vi "StageLinear.vi"(0 "Axis":T1={"Serial port handle"="", "Axis"="", "Controller #"=0, "Min position"=0.0, "Max position"=0.0, "Min velocity"=0.0, "Max velocity"=0.0, "Firmware"="", "Device ID"=0, "Variable event"=refnum, "Variable ref"=refnum, "Resolution, usteps/step"=0, "Serial port semaphore"=refnum, "Joystick buttons"={"MinDir"=1, "MaxDir"=2, "MedSpeed"=5, "HighSpeed"=6}} {"Joystick buttons"."HighSpeed" min=1 max=25 step=1; "Joystick buttons"."MedSpeed" min=1 max=25 step=1; "Joystick buttons"."MaxDir" min=1 max=25 step=1; "Joystick buttons"."MinDir" min=1 max=25 step=1}, 2 "Joystick event":T4, 3 "Stop event":refnum<user-event>, 5 "error in":errorcluster={"status"=FALSE, "code"=1073676294, "source"="VISA Read in Zaber TLCM.lvclass:Command.vi:1820008->Zaber TLCM.lvclass:Get home position.vi->Zaber TLCM.lvclass:Get limits.vi->Zaber TLCM.lvclass:Join.vi->Swan probe.vi"}) -> (14 "Axis out":T1={"Serial port handle"="", "Axis"="", "Controller #"=0, "Min position"=0.0, "Max position"=0.0, "Min velocity"=0.0, "Max velocity"=0.0, "Firmware"="", "Device ID"=0, "Variable event"=refnum, "Variable ref"=refnum, "Resolution, usteps/step"=0, "Serial port semaphore"=refnum, "Joystick buttons"={"MinDir"=1, "MaxDir"=2, "MedSpeed"=5, "HighSpeed"=6}} {"Joystick buttons"."HighSpeed" min=1 max=25 step=1; "Joystick buttons"."MedSpeed" min=1 max=25 step=1; "Joystick buttons"."MaxDir" min=1 max=25 step=1; "Joystick buttons"."MinDir" min=1 max=25 step=1}, 19 "error out":errorcluster)   [LabVIEW 2017]
uses:
  Joystick events/Joystick event.ctl
  GenericDataEvent/GenericEvent.ctl
  Zaber.ctl
  ZaberVariables.ctl
panel:
  in  "Tab Control":enum32{"Joystick", "Keyboard"}(tab)
  in  "JoyLowVel":dbl=0.02 caption="Low velocity, mm/s" min=1e-07 max=25.0 step=0.01 format="%#.4f"
  in  "JoyMediumVel":dbl=1.0 caption="Medium velocity, mm/s" min=1e-07 max=25.0 step=0.01 format="%#.4f"
  in  "JoyHighVel":dbl=5.0 caption="High velocity, mm/s" min=1e-07 max=25.0 step=0.01 format="%#.4f"
  out "JoyMinDirection":i32=1 caption="Min direction" min=1 max=25 step=1
  out "JoyMaxDirection":i32=2 caption="Max direction" min=1 max=25 step=1
  out "JoyMediumVelocity":i32=5 caption="Max direction" min=1 max=25 step=1
  out "JoyHighVelocity":i32=6 caption="Max direction" min=1 max=25 step=1
  in  "BtnJogNegative":bool
  in  "BtnJogPositive":bool
  in  "JogStep":dbl=0.02 caption="Jog step, mm" min=1e-07 max=25.0 step=0.01 format="%#.4f"
  out "JoystickValue":i16
  in  "Readback loop":bool=TRUE
  out "Name":string
  in  "VelocitySp":dbl=0.19998779296875002 caption="Velocity, mm/s" min=0.0 max=25.40003175 format="%#.6f"
  out "VelocityRb":dbl=0.19998779296875002 caption="X position" min=0.0 max=25.0 format="%#.6f"
  in  "PositionSp":dbl caption="Position, mm" min=0.0 max=25.40003175 format="%#.6f"
  out "PositionRb":dbl=0.8111490000000001 caption="X position" min=0.0 max=25.0 format="%#.6f"
  out "MaxVelocity":dbl=26.0 caption="Max velocity, mm/s" format="%#.4f"
  out "MaxPositionRb":dbl=101.60003175000001 caption="Max position, mm" format="%#.4f"
  out "MinPositionRb":dbl caption="Min position, mm" format="%#.4f"
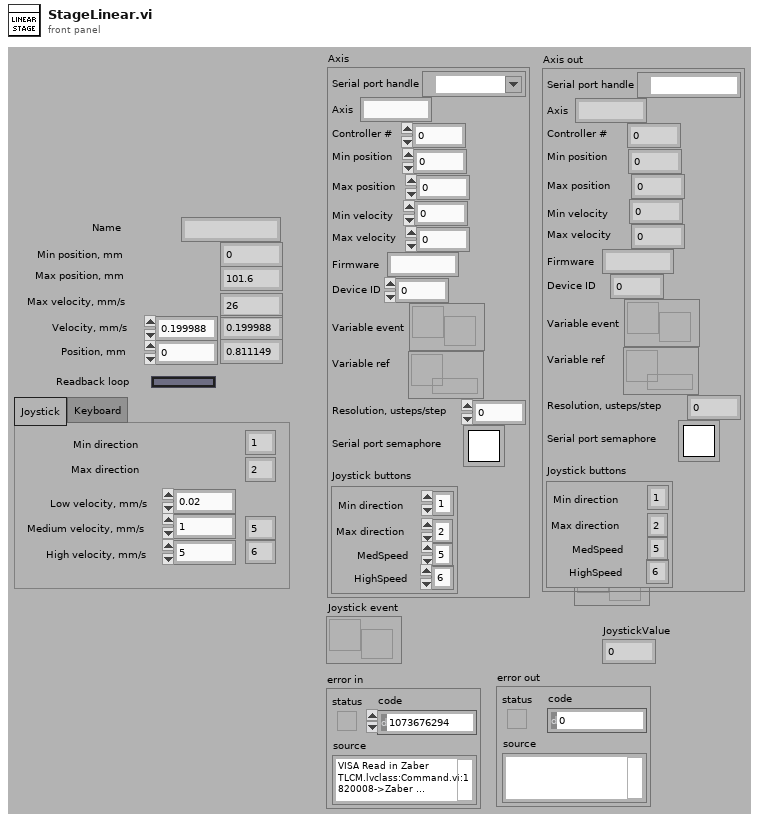
[diagram p1: front panel]
types:
  T1 = typedef "Zaber.ctl" = cluster{"Serial port handle":refnum<visa-resource-name>, "Axis":string, "Controller #":u8, "Min position":dbl, "Max position":dbl, "Min velocity":dbl, "Max velocity":dbl, "Firmware":string, "Device ID":i32, "Variable event":T2, "Variable ref":refnum<data-value>, "Resolution, usteps/step":i32, "Serial port semaphore":T3, "Joystick buttons":cluster{"MinDir":i32, "MaxDir":i32, "MedSpeed":i32, "HighSpeed":i32}}
  T2 = typedef "GenericEvent.ctl" = refnum<user-event>
  T3 = typedef "Semaphore RefNum" = refnum<k1>
  T4 = typedef "Joystick event.ctl" = refnum<user-event>
  T5 = cluster{"MinDir":i32, "MaxDir":i32, "MedSpeed":i32, "HighSpeed":i32}
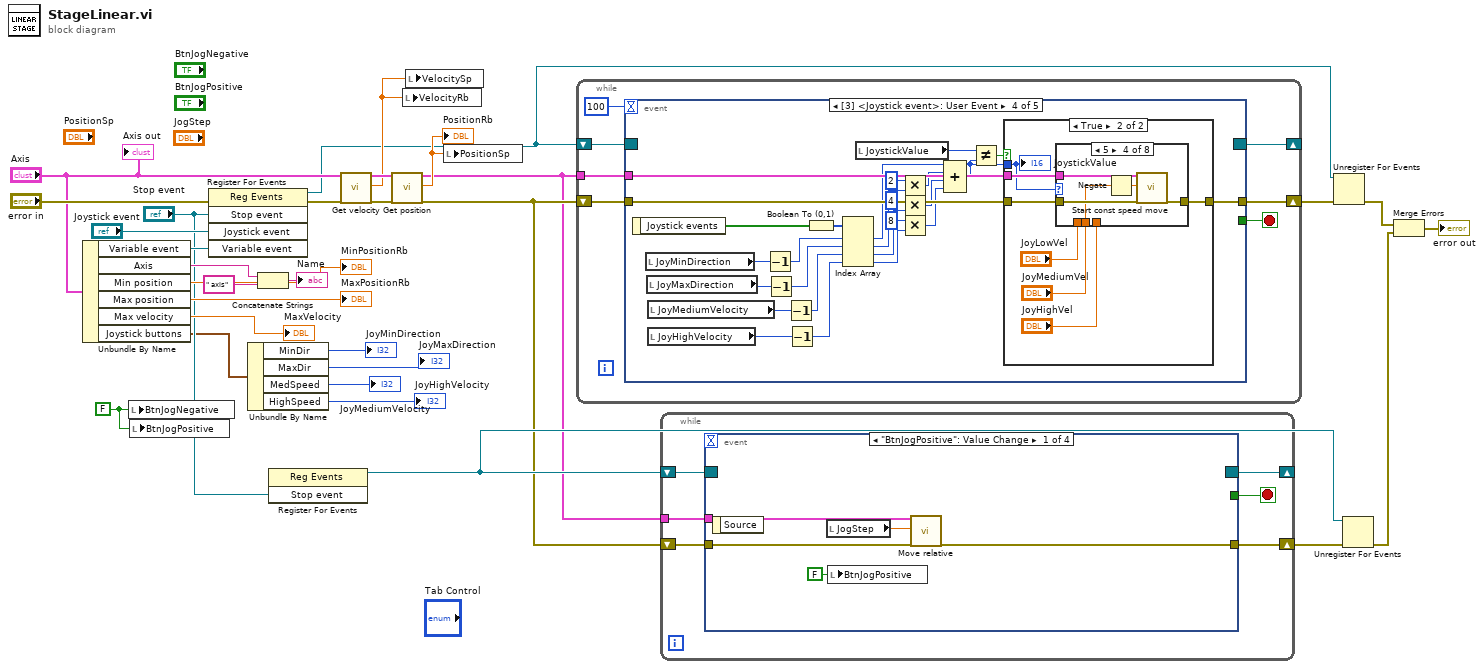
[diagram p0: block diagram]
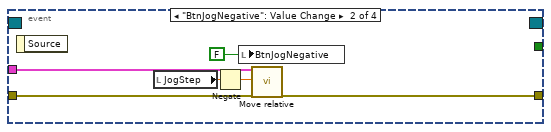
[diagram p2: hidden frame]
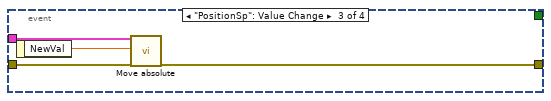
[diagram p3: hidden frame]
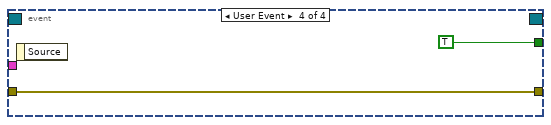
[diagram p4: hidden frame]
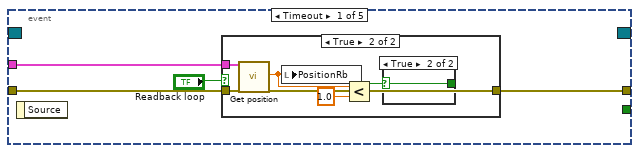
[diagram p5: hidden frame]
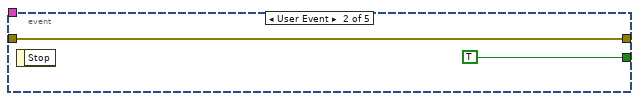
[diagram p8: hidden frame]
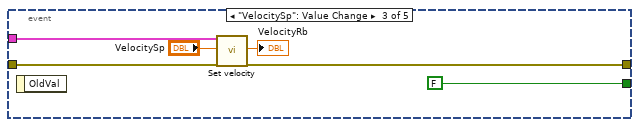
[diagram p9: hidden frame]
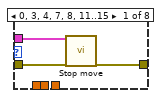
[diagram p11: hidden frame]
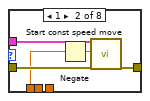
[diagram p12: hidden frame]
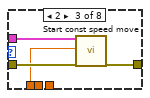
[diagram p13: hidden frame]
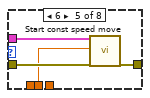
[diagram p14: hidden frame]
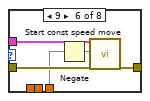
[diagram p15: hidden frame]
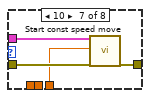
[diagram p16: hidden frame]
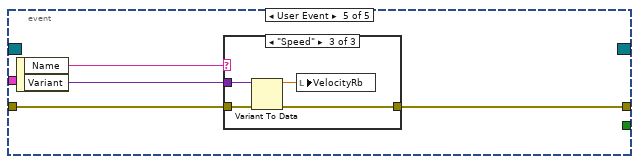
[diagram p18: hidden frame]
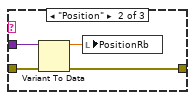
[diagram p20: hidden frame]
diagram:
  w30 = FALSE
  n1 = Unbundle By Name("Axis") -> ("Variable event"=w27:T2, "Axis"=w25:string, "Min position"=→"MinPositionRb":dbl, "Max position"=→"MaxPositionRb":dbl, "Max velocity"=→"MaxVelocity":dbl, "Joystick buttons"=w7:T5)
  n2 = local write "BtnJogNegative"(w30) -> ()
  n3 = local write "BtnJogPositive"(w30) -> ()
  n4 = register-events(error in="error in", "Stop event", "Joystick event", w27) -> (reference out=w15:refnum<event-registration>, error out=w19:errorcluster)  [unwired: 1 in]
  n5 = Unbundle By Name(w7) -> ("MinDir"=→"JoyMinDirection":i32, "MaxDir"=→"JoyMaxDirection":i32, "MedSpeed"=→"JoyMediumVelocity":i32, "HighSpeed"=→"JoyHighVelocity":i32)
  n6 = Concatenate Strings(w25, " axis" ("string")) -> (→"Name":string)
  n7 = register-events("Stop event") -> (reference out=w13:refnum<event-registration>)  [unwired: 2 in, 1 out]
  n8 = call "Get velocity.vi"("Zaber"="Axis", "error in"=w19) -> ("Zaber out"=w23:T1, "Velocity, mm/s"=w22:dbl, "error out"=w31:errorcluster)  [unwired: 14 in, 1 out]
  n9 = call "Get position.vi"("Zaber"=w23, "error in"=w31) -> ("Zaber out"=w5:T1, "PositionRb"=w21:dbl, "error out"=w6:errorcluster)  [unwired: 13 in, 2 out]
  "PositionRb" <- w21
  n10 = local write "VelocityRb"(w22) -> ()
  n11 = local write "VelocitySp"(w22) -> ()
  n12 = local write "PositionSp"(w21) -> ()
  n13 = while {
    shift-right: [w35] -> w11
    shift-left: w6 -> [w36]
    tunnel: w5 -> [w37]
    shift-right: [w32] -> _
    shift-left: w15 -> [w34]
    stop <- w38 stop-if-true
    n14 = event shown="[3] <Joystick event>: User Event" {
      selector: w34 -> [_ _ _ _ _]
      dyn-events: [_ _ _ _ _] -> w32
      timeout: 100 -> [_ _ _ _ _]
      tunnel: [_ TRUE ("Stop") FALSE ("Stop") _ _] -> w38
      tunnel: w36 -> [w40 w52 w58 w82 w127]
      tunnel: w37 -> [w41 _ w53 w81 _]
      tunnel: [w39 w52 w55 w80 w126] -> w35
      event Timeout {
        n15 = event-data() -> ()  [unwired: 2 out]
        n16 = case shown="True" "Readback loop" {
          tunnel: w40 -> [w43 w49]
          tunnel: w41 -> [_ w47]
          tunnel: [w43 w48] -> w39
          frame False {
          }
          frame True {
            n17 = call "Get position.vi"("Zaber"=w47, "error in"=w49) -> ("PositionRb"=w46:dbl, "error out"=w48:errorcluster)  [unwired: 13 in, 3 out]
            n18 = local write "PositionRb"(w46) -> ()
            n19 = Less?(x=w46, y=1.0) -> (x < y?=w44:bool)
            n20 = case shown="True" w44 {
              selector: w44 -> [_ w50]
              tunnel: [_ w50] -> _
              frame False {
              }
              frame True {
              }
            }
          }
        }
      }
      event User Event {
        n21 = event-data() -> ()  [unwired: 2 out]
      }
      event "VelocitySp": Value Change {
        n22 = event-data() -> ()  [unwired: 2 out]
        n23 = call "Set velocity.vi"("Zaber in"=w53, "Velocity, mm/s"="VelocitySp", "error in"=w58) -> ("Velocity, mm/s"=→"VelocityRb":dbl, "error out"=w55:errorcluster)  [unwired: 14 in, 1 out]
      }
      event User Event {
        n24 = event-data() -> ("Joystick events"=w84:bool[])  [unwired: 1 out]
        n25 = local read "JoyMinDirection"() -> (w62:i32)
        n26 = local read "JoyMaxDirection"() -> (w61:i32)
        n27 = local read "JoyMediumVelocity"() -> (w60:i32)
        n28 = local read "JoyHighVelocity"() -> (w59:i32)
        n29 = Decrement(x=w62) -> (x-1=w79:i32)
        n30 = Decrement(x=w61) -> (x-1=w78:i32)
        n31 = Decrement(x=w60) -> (x-1=w77:i32)
        n32 = Decrement(x=w59) -> (x-1=w76:i32)
        n33 = Boolean To (0,1)(Boolean=w84) -> (0, 1=w83:i16[])
        n34 = Index Array(array=w83, index #1=w79, index #2=w78, index #3=w77, index #4=w76) -> (element #1=w70:i16, element #2=w63:i16, element #3=w74:i16, element #4=w72:i16)
        n35 = local read "JoystickValue"() -> (w66:i16)
        n36 = Multiply(x=i16 2 ("y"), y=w63) -> (x*y=w69:i16)
        n37 = Multiply(x=i16 4 ("y"), y=w74) -> (x*y=w68:i16)
        n38 = Multiply(x=i16 8 ("y"), y=w72) -> (x*y=w67:i16)
        n39 = Compound Arithmetic op=ADD(w70, w69, w68, w67) -> (w64:i16)
        n40 = Not Equal?(x=w66, y=w64) -> (x != y?=w65:bool)
        n41 = case shown="True" w65 {
          tunnel: w82 -> [w85 w92]
          tunnel: w81 -> [_ w91]
          tunnel: [w85 w90] -> w80
          tunnel: w64 -> [_ w89]
          frame False {
          }
          frame True {
            n42 = case shown="5" w89 {
              tunnel: w92 -> [w95 w98 w102 w107 w111 w116 w120 w123]
              tunnel: w91 -> [w94 w99 w103 w108 w112 w117 w121 _]
              tunnel: [w93 w100 w104 w109 w113 w118 w122 w123] -> w90
              tunnel: "JoyLowVel" -> [_ w96 w101 _ _ _ _ _]
              tunnel: "JoyMediumVel" -> [_ _ _ w105 w110 _ _ _]
              tunnel: "JoyHighVel" -> [_ _ _ _ _ w114 w119 _]
              frame 0, 3, 4, 7, 8, 11..15 {
                n43 = call "Stop move.vi"("Zaber"=w94, "error in"=w95) -> ("error out"=w93:errorcluster)  [unwired: 16 in, 1 out]
              }
              frame 1 {
                n44 = Negate(x=w96) -> (-x=w97:dbl)
                n45 = call "Start const speed move.vi"("Zaber"=w99, "Velocity, mm/s"=w97, "error in"=w98) -> ("error out"=w100:errorcluster)  [unwired: 14 in, 2 out]
              }
              frame 2 {
                n46 = call "Start const speed move.vi"("Zaber"=w103, "Velocity, mm/s"=w101, "error in"=w102) -> ("error out"=w104:errorcluster)  [unwired: 14 in, 2 out]
              }
              frame 5 {
                n47 = Negate(x=w105) -> (-x=w106:dbl)
                n48 = call "Start const speed move.vi"("Zaber"=w108, "Velocity, mm/s"=w106, "error in"=w107) -> ("error out"=w109:errorcluster)  [unwired: 14 in, 2 out]
              }
              frame 6 {
                n49 = call "Start const speed move.vi"("Zaber"=w112, "Velocity, mm/s"=w110, "error in"=w111) -> ("error out"=w113:errorcluster)  [unwired: 14 in, 2 out]
              }
              frame 9 {
                n50 = Negate(x=w114) -> (-x=w115:dbl)
                n51 = call "Start const speed move.vi"("Zaber"=w117, "Velocity, mm/s"=w115, "error in"=w116) -> ("error out"=w118:errorcluster)  [unwired: 14 in, 2 out]
              }
              frame 10 {
                n52 = call "Start const speed move.vi"("Zaber"=w121, "Velocity, mm/s"=w119, "error in"=w120) -> ("error out"=w122:errorcluster)  [unwired: 14 in, 2 out]
              }
              frame Default {
              }
            }
            "JoystickValue" <- w89
          }
        }
      }
      event User Event {
        n53 = event-data() -> ("Name"=w125:string, "Variant"=w124:variant)  [unwired: 1 out]
        n54 = case shown="\"Speed\"" w125 {
          tunnel: w124 -> [_ w132 w135]
          tunnel: w127 -> [w128 w131 w136]
          tunnel: [w128 w130 w134] -> w126
          frame Default {
          }
          frame "Position" {
            n55 = Variant To Data(error in=w131, Variant=w132) -> (data=w129:dbl, error out=w130:errorcluster)  [unwired: 1 in]
            n56 = local write "PositionRb"(w129) -> ()
          }
          frame "Speed" {
            n57 = Variant To Data(error in=w136, Variant=w135) -> (data=w133:dbl, error out=w134:errorcluster)  [unwired: 1 in]
            n58 = local write "VelocityRb"(w133) -> ()
          }
        }
      }
    }
  }
  n59 = while {
    shift-right: [w141] -> w12
    shift-left: w6 -> [w142]
    tunnel: w5 -> [w140]
    shift-right: [w137] -> _
    shift-left: w13 -> [w139]
    stop <- w138 stop-if-true
    n60 = event shown="[0] \"BtnJogPositive\": Value Change" {
      selector: w139 -> [_ _ _ _]
      dyn-events: [_ _ _ _] -> w137
      timeout: _ -> [_ _ _ _]
      tunnel: w142 -> [w145 w150 w157 w158]
      tunnel: [w143 w149 w156 w158] -> w141
      tunnel: w140 -> [w144 w148 w155 _]
      tunnel: [_ _ _ TRUE ("Stop")] -> w138
      event "BtnJogPositive": Value Change {
        n61 = event-data() -> ()  [unwired: 1 in, 1 out]
        n62 = local read "JogStep"() -> (w147:dbl)
        n63 = local write "BtnJogPositive"(FALSE) -> ()
        n64 = call "Move relative.vi"("Zaber"=w144, "Distance, mm"=w147, "error in"=w145) -> ("error out"=w143:errorcluster)  [unwired: 13 in, 3 out]
      }
      event "BtnJogNegative": Value Change {
        n65 = event-data() -> ()  [unwired: 1 in, 1 out]
        n66 = local read "JogStep"() -> (w153:dbl)
        n67 = Negate(x=w153) -> (-x=w152:dbl)
        n68 = local write "BtnJogNegative"(FALSE) -> ()
        n69 = call "Move relative.vi"("Zaber"=w148, "Distance, mm"=w152, "error in"=w150) -> ("error out"=w149:errorcluster)  [unwired: 13 in, 3 out]
      }
      event "PositionSp": Value Change {
        n70 = event-data() -> ("NewVal"=w154:dbl)  [unwired: 1 in]
        n71 = call "Move absolute.vi"("Zaber"=w155, "Position, mm"=w154, "error in"=w157) -> ("error out"=w156:errorcluster)  [unwired: 13 in, 3 out]
      }
      event User Event {
        n72 = event-data() -> ()  [unwired: 1 in, 1 out]
      }
    }
  }
  n73 = Unregister For Events(event registration refnum=w15, error in=w11) -> (error out=w9:errorcluster)
  n74 = Unregister For Events(event registration refnum=w13, error in=w12) -> (error out=w10:errorcluster)
  n75 = Merge Errors(w9, w10) -> (→"error out":errorcluster)
  "Axis out" <- "Axis"
